vi "Limit Lines.vi"(8 "error in (no error)":errorcluster, 10 "Count":i32, 11 "TermBuffer in":refnum<class "TermBuffer.lvclass">) -> (0 "error out":errorcluster, 3 "TermBuffer out":refnum<class "TermBuffer.lvclass">)   [LabVIEW 2020, in "Terminal.lvlib" / "TermBuffer.lvclass"]
uses:
  TermBuffer.lvclass
  TermBuffer.lvclass/TermBuffer.ctl
  TermLine/TermLine.lvclass
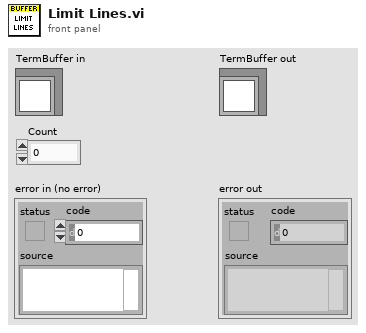
[diagram p1: front panel]
types:
  T1 = typedef "Terminal.lvlib/TermBuffer.lvclass/Ref Data.ctl" = cluster{"Lines":refnum<class "TermLine.lvclass">[], "Rows":i32, "Cols":i32}
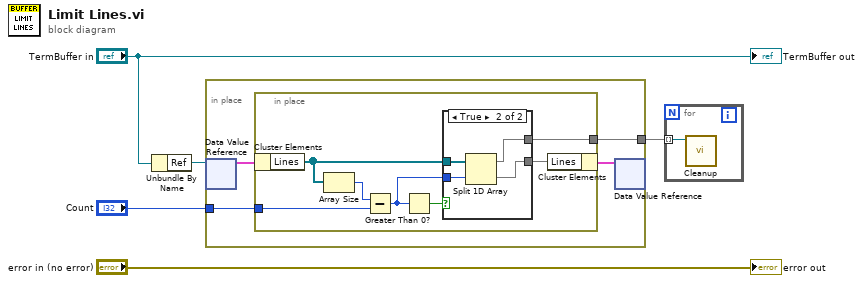
[diagram p0: block diagram]
diagram:
  n1 = Unbundle By Name("TermBuffer in") -> ("Ref"=w4:refnum<data-value>)
  n2 = in-place {
    in-place-border: [w7] -> w2
    in-place-border: "Count" -> [w6]
    n3 = in-place-dvr #1(w4) -> (w9:T1)  [unwired: 1 out]
    n4 = in-place {
      in-place-border: [w15] -> w7
      in-place-border: w6 -> [w13]
      n5 = in-place-cluster #2(w9) -> ("Lines"=w14:refnum<class "TermLine.lvclass">[])
      n6 = Array Size(array=w14) -> (size(s)=w12:i32)
      n7 = Subtract(x=w12, y=w13) -> (x-y=w11:i32)
      n8 = Greater Than 0?(x=w11) -> (x > 0?=w10:bool)
      n9 = case shown="True" w10 {
        tunnel: [w17 w21] -> w16
        tunnel: [_ w20] -> w15
        tunnel: w14 -> [w17 w19]
        tunnel: w11 -> [_ w18]
        frame False {
        }
        frame True {
          n10 = Split 1D Array(array=w19, index=w18) -> (first subarray=w20:refnum<class "TermLine.lvclass">[], second subarray=w21:refnum<class "TermLine.lvclass">[])
        }
      }
      n11 = in-place-cluster #2("Lines"=w16) -> (w8:T1)
    }
    n12 = in-place-dvr #1(w8) -> ()  [unwired: 2 out]
  }
  n13 = for {
    tunnel: w2 -> [w22] mode=indexing
    n14 = call "Cleanup.vi"("TermLine in"=w22) -> ()  [unwired: 10 in, 1 out]
  }
  "error out" <- "error in (no error)"
  "TermBuffer out" <- "TermBuffer in"
